vi "字符串数组拼接.vi"(11 "数组":string[](array[string])) -> (3 "字符串":string)   [LabVIEW 2019]
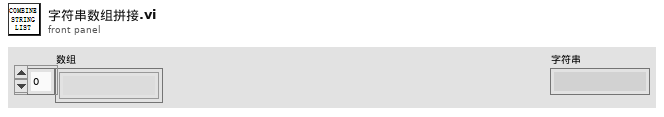
[diagram p1: front panel]
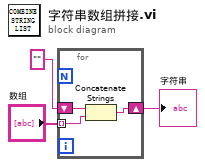
[diagram p0: block diagram]
diagram:
  n1 = for {
    tunnel: "数组" -> [w6] mode=indexing
    shift-right: [w5] -> w1
    shift-left: "" -> [w4]
    n2 = Concatenate Strings(w4, w6) -> (w5:string)
  }
  "字符串" <- w1
